vi "LED Config-3Colors.vi"(8 "refnum name":string, 9 "Channel C":bool, 10 "Channel B":bool, 11 "Channel A":bool) -> ()   [LabVIEW 2019]
uses:
  <vilib>/Rock Robotics/WPI/ThirdParty/Phoenix-LabVIEW/CANifier/CTRE_CANifier_LEDChannel.ctl
  mOS_XIII/MoS_XIII/Globals/LED_Globals.vi
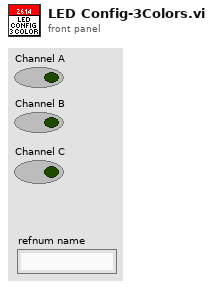
[diagram p1: front panel]
types:
  T1 = typedef "CTRE_CANifier_LEDChannel.ctl" = enum32{"LEDChannelA", "LEDChannelB", "LEDChannelC"}
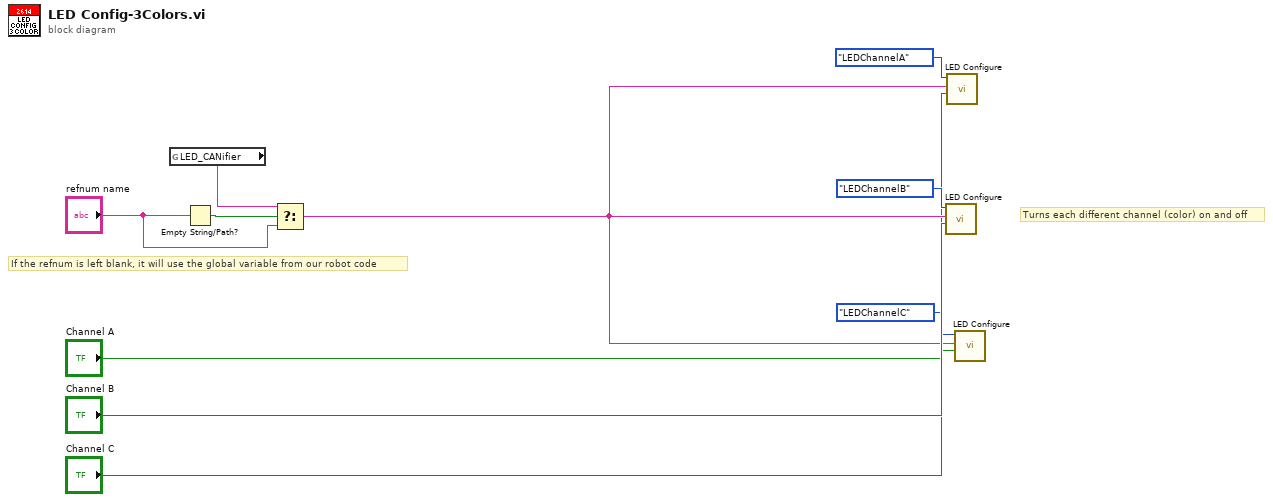
[diagram p0: block diagram]
diagram:
  # "Turns each different channel (color) on and off"
  # "If the refnum is left blank, it will use the global variable from our robot code"
  n1 = global read "LED_Globals.vi" "LED_CANifier"() -> (w4:string)
  n2 = Empty String/Path?(string/path="refnum name") -> (empty?=w5:bool)
  n3 = Select(t=w4, s=w5, f="refnum name") -> (s? t:f=w2:string)
  n4 = call "LED Configure.vi"("LED On"="Channel B", "refnum name"=w2, "LEDChannel"=CTRE_CANifier_LEDChannel."LEDChannelB") -> ()  [unwired: 9 in]
  n5 = call "LED Configure.vi"("LED On"="Channel A", "refnum name"=w2, "LEDChannel"=CTRE_CANifier_LEDChannel."LEDChannelA") -> ()  [unwired: 9 in]
  n6 = call "LED Configure.vi"("LED On"="Channel C", "refnum name"=w2, "LEDChannel"=CTRE_CANifier_LEDChannel."LEDChannelC") -> ()  [unwired: 9 in]
